vi "Global_SM Write_Data Out.vi"() -> ()   [LabVIEW 2017, in "Claw.lvlib"]
uses:
  startup.rtexe/Claw.lvlib
  startup.rtexe/WPI_SolenoidValue.ctl
  startup.rtexe/CLUSTER_Two Motor Input.ctl
panel:
  in  "Claw_SM_Motor_Input":T1
  in  "Claw_SM_Pistion_Input":T2
  # "The Names of the Data items in the Global Variable MUST describe who the Single Writer is\nNaming Convention of all Data Items is:   \nLib Name_Loop Name (SM or SEN or ACT)_Data Name\nExamples:\nDrive_ACT_X axis\nGameController_SEN_JoystickLeft\nHopper_SM_AgitatorSpeed"
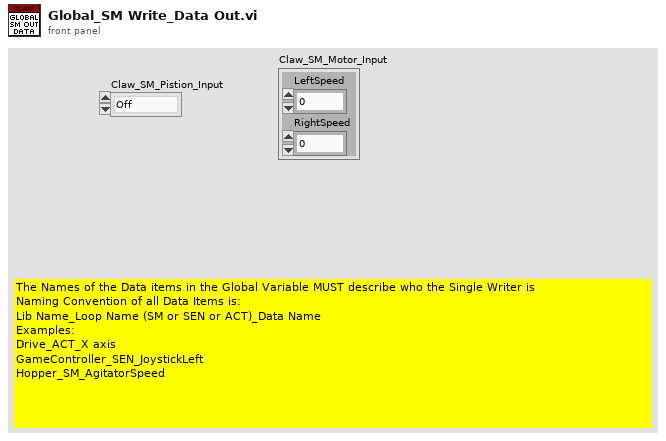
[diagram p1: front panel]
types:
  T1 = typedef "CLUSTER_Two Motor Input.ctl" = cluster{"LeftSpeed":dbl, "RightSpeed":dbl}
  T2 = typedef "WPI_SolenoidValue.ctl" = enum16{"Off", "On", "Forward", "Reverse"}
diagram:
